vi "CloseFpga.vi"(8 "error in (no error)":errorcluster, 11 "FpgaInterface in":refnum<class "FpgaInterface.lvclass">) -> (0 "error out":errorcluster, 3 "FpgaInterface out":refnum<class "FpgaInterface.lvclass">)   [LabVIEW 2017, in "FpgaInterface.lvclass"]
uses:
  FpgaInterface.lvclass
  FpgaInterface.lvclass/FpgaInterface.ctl
  <vilib>/FPGAPlugInAG/Dynamic/niLvFpga_Close_Dynamic.vi
  <vilib>/rvi/interface/nirviCloseFPGA/nirviCloseFPGA.xnode
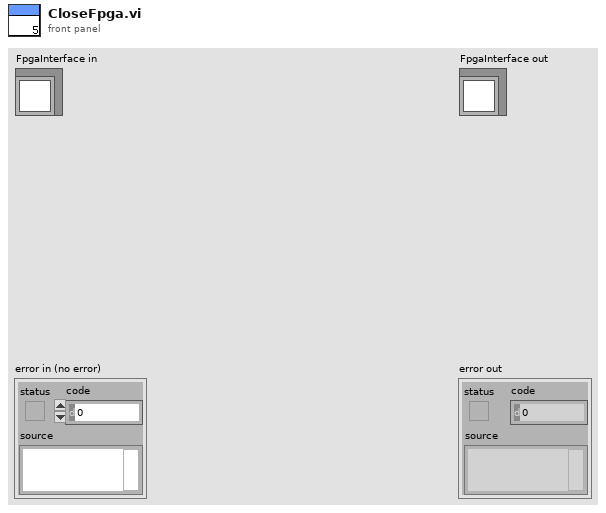
[diagram p1: front panel]
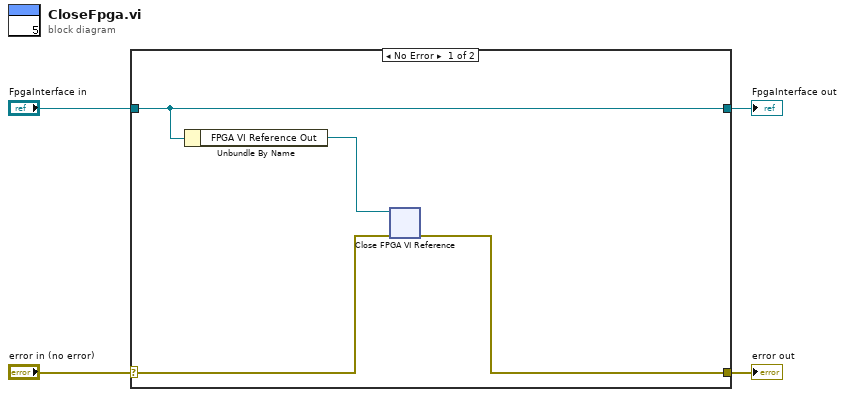
[diagram p0: block diagram]
diagram:
  n1 = case shown="No Error" "error in (no error)" {
    selector: "error in (no error)" -> [w8 w10]
    tunnel: [w7 w10] -> w3
    tunnel: [w6 w9] -> w1
    tunnel: "FpgaInterface in" -> [w6 w9]
    frame No Error {
      n2 = Unbundle By Name(w6) -> ("FPGA VI Reference Out"=w5:refnum<k20>)
      n3 = xnode "Close FPGA VI Reference"("FPGA VI Reference In"=w5, "error in"=w8) -> ("error out"=w7:errorcluster)
    }
    frame Error {
    }
  }
  "error out" <- w3
  "FpgaInterface out" <- w1
